vi "DefaultFromINI.vi"(8 "error in (no error)":errorcluster, 11 "NHRDCPower":refnum<class "NHRDCPower.lvclass">) -> (0 "error out":errorcluster, 3 "NHRDCPower":refnum<class "NHRDCPower.lvclass">)   [LabVIEW 2018, in "AcPwrPlugins.lvlib" / "NHRDCPower.lvclass"]
doc: "This VI reads the current configuration stored in the INI file."
uses:
  NHRDCPower.lvclass
  C:/Program Files (x86)/National Instruments/LabVIEW 2018/user.lib/NIST/BaseClasses/BasePlugin_class/BasePlugin.lvclass
  C:/Users/ico/Documents/Projects/NistPluggableModules/AcPwr/AcPwrPlugins/AcPwrBaseClass/AcPwrBase.lvclass
  TypeDefs/Measurements.ctl
  TypeDefs/Device(s)Settings.ctl
  TypeDefs/Modules.ctl
  <userlib>/NIST/BaseClasses/BasePlugin_class/BasePlugin.lvclass/BasePlugin.ctl
  <userlib>/NIST/BaseClasses/BasePlugin_class/Accessors/Read PluginIniFilePath.vi
  AcPwrBaseClass/AcPwrBase.lvclass
  <vilib>/Utility/config.llb/NI_LVConfig.lvlib
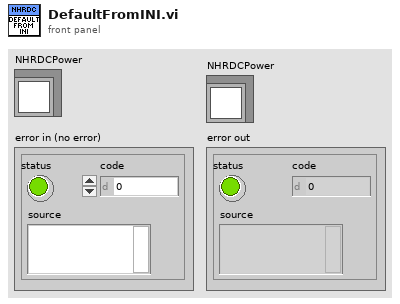
[diagram p1: front panel]
types:
  T1 = typedef "AcPwrPlugins.lvlib/NHRDCPower.lvclass/Device(s)Settings.ctl" = cluster{"MeasName":string, "Modules":T2}
  T2 = typedef "AcPwrPlugins.lvlib/NHRDCPower.lvclass/Modules.ctl" = cluster{"Handle":string, "Name":string, "id query (Yes)":bool, "reset device (Yes)":bool, "Connected":bool, "Initial Battery Detect Voltage (0)":dbl, "SafetySettings":cluster{"SetWatchDog?":bool, "Voltage (V)":dbl, "Current (A)":dbl, "Power (W)":dbl, "Voltage Delay (s)":dbl, "Current Delay (s)":dbl, "Power Delay (s)":dbl}, "Options String":string, "Aperture Time (s)":dbl, "operating state (Off)":i32, "OutputSettings":cluster{"Voltage (V)":dbl, "Current (A)":dbl, "Resistance (Ohms)":dbl, "Power (W)":dbl, "Enable Voltage":bool, "Enable Current":bool, "Enable Resistance":bool, "Enable Power":bool, "Macro After Step Delay  (s)":dbl, "Wait Value (V, A, W)":dbl, "Enable Wait":bool, "Wait on Value":i32}[], "SlewRate":cluster{"Set Voltage Rate V/S":dbl, "Set Current Rate A/S":dbl, "Set Resistance Rate R/S":dbl, "Set Power Rate W/S":dbl}, "Macro":cluster{"Save Macro?":bool, "Load Macro From File?":bool, "Run Macro Continuously?":bool, "Use Macros?":bool, "Load Macro File Path":string, "Save Macro File Path":string}, "Regulation Gain (1=100%)":dbl, "UpdatingOntheFly":bool}[]
  T3 = typedef "AcPwrPlugins.lvlib/NHRDCPower.lvclass/Measurements.ctl" = cluster{"Handle":string, "Name":string, "Enabled":bool, "Measurement Value":sgl, "Measurement Type":enum16{"Power", "Current", "Voltage"}}[]
  T4 = typedef "NI_LVConfig.lvlib/Config Data RefNum.ctl" = refnum<k1>
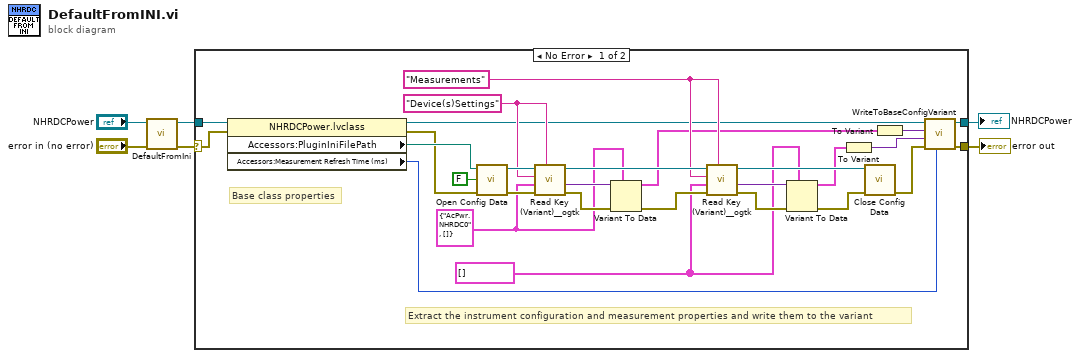
[diagram p0: block diagram]
diagram:
  n1 = call-parent "DefaultFromIni.vi"("error in (no error)"="error in (no error)", "AcPwrBase"="NHRDCPower") -> ("error out"=w6:errorcluster, "AcPwrBase"=w5:refnum<class "NHRDCPower.lvclass">)  [unwired: 8 in]
  n2 = case shown="No Error" w6 {
    selector: w6 -> [w8 w35]
    tunnel: w5 -> [w9 w36]
    tunnel: [w16 w36] -> w2
    tunnel: [w18 w35] -> w1
    frame No Error {
      w12 = T1 {"MeasName"="AcPwr.NHRDC0", "Modules"=[]} ("NHRDC")
      w19 = T3 [] ("Measurements")
      w20 = "Measurements" ("section")
      w28 = "Device(s)Settings" ("section")
      # "Extract the instrument configuration and measurement properties and write them to the variant"
      # "Base class properties"
      n3 = property class="NHRDCPower.lvclass"(reference=w9, error in=w8) -> (reference out=w13:refnum<class "NHRDCPower.lvclass">, error out=w27:errorcluster, "Accessors:PluginIniFilePath"=w34:path, "Accessors:Measurement Refresh Time (ms)"=w7:u32)
      n4 = call <vilib>:"Open Config Data.vi"("error in (no error)"=w27, "create file if necessary (T)"=FALSE, "configuration file path"=w34) -> ("error out"=w31:errorcluster, "refnum"=w32:T4)  [unwired: 6 in, 1 out]
      n5 = call <userlib>:"Read Key (Variant)__ogtk.vi"("section"=w28, "error in (no error)"=w31, "type"=w12, "key (optional)"=w28, "refnum"=w32) -> ("error out"=w29:errorcluster, "key-value"=w30:variant, "refnum out"=w24:T4)  [unwired: 3 in, 1 out]
      n6 = Variant To Data(error in=w29, type=w12, Variant=w30) -> (data=w14:T1, error out=w21:errorcluster)
      n7 = call <userlib>:"Read Key (Variant)__ogtk.vi"("section"=w20, "error in (no error)"=w21, "type"=w19, "key (optional)"=w20, "refnum"=w24) -> ("error out"=w26:errorcluster, "key-value"=w25:variant, "refnum out"=w23:T4)  [unwired: 3 in, 1 out]
      n8 = Variant To Data(error in=w26, type=w19, Variant=w25) -> (data=w10:T3, error out=w22:errorcluster)
      n9 = To Variant(anything=w10) -> (Variant=w11:variant)
      n10 = call <vilib>:"Close Config Data.vi"("error in (no error)"=w22, "refnum"=w23) -> ("error out"=w17:errorcluster)  [unwired: 8 in, 1 out]
      n11 = To Variant(anything=w14) -> (Variant=w15:variant)
      n12 = call "WriteToBaseConfigVariant.vi"("Measurement Refresh Time (ms)"=w7, "error in (no error)"=w17, "Meas"=w11, "Config"=w15, "NHRDCPower in"=w13) -> ("error out"=w18:errorcluster, "NHRDCPower out"=w16:refnum<class "NHRDCPower.lvclass">)  [unwired: 5 in]
    }
    frame Error {
    }
  }
  "error out" <- w1
  "NHRDCPower" <- w2
